vi "Test 2.vi"() -> ()   [LabVIEW 2019]
panel:
  in  "Sample Rate":fxp<+,12,12>
  in  "Ready":bool
  out "Increment":bool
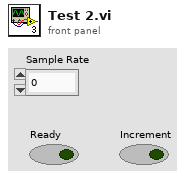
[diagram p1: front panel]
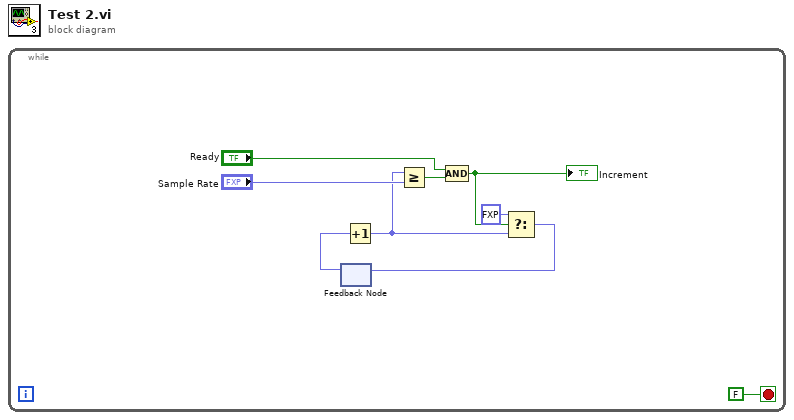
[diagram p0: block diagram]
diagram:
  n1 = while {
    stop <- FALSE stop-if-true
    n2 = feedback #1() -> (w3:fxp<+,12,12>)  [unwired: 1 in]
    n3 = Increment(x=w3) -> (x+1=w2:fxp<+,12,12>)
    n4 = Greater Or Equal?(x=w2, y="Sample Rate") -> (x >= y?=w7:bool)
    n5 = Compound Arithmetic op=AND("Ready", w7) -> (w5:bool)
    "Increment" <- w5
    n6 = Select(t=fxp<+,12,12> 0.0, s=w5, f=w2) -> (s? t:f=w8:fxp<+,12,12>)
    n7 = feedback-in #1(w8) -> ()
  }
